vi "Prob.vi"(1 "Data":string[][](array[string])) -> (0 "Success %":dbl, 2 "Histogram_Speed":T1(graph), 3 "Histogram_Length":T1(graph), 4 "E[Speed]":dbl format="%0.2f", 5 "Var[Speed]":dbl format="%0.2f", 6 "E[Length]":dbl format="%0.2f", 7 "Var[Length]":dbl format="%0.2f")   [LabVIEW 2020]
uses:
  <vilib>/Analysis/NI_AALBase.lvlib
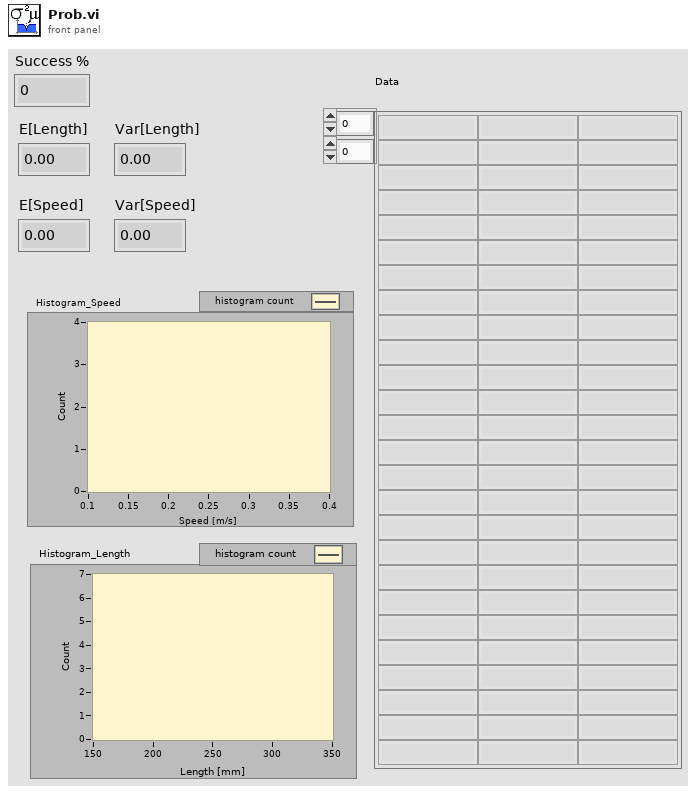
[diagram p1: front panel]
types:
  T1 = cluster{"X Values":dbl[], "Histogram: h(x)":i32[]}
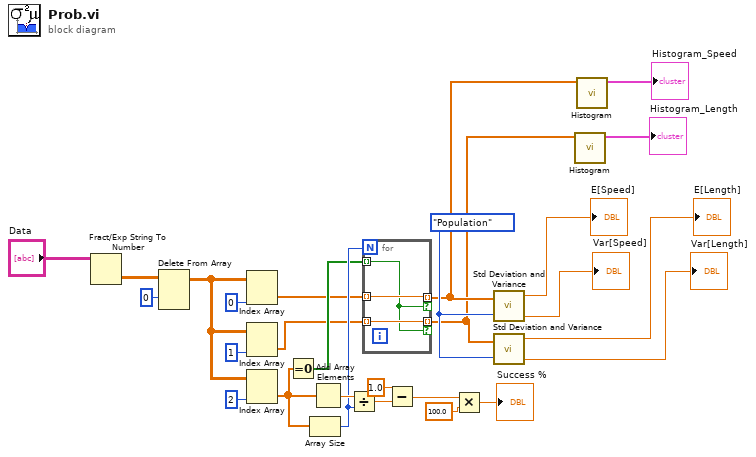
[diagram p0: block diagram]
diagram:
  w7 = enum16{"Sample", "Population"}."Population" ("Weighting (Sample)")
  n1 = Fract/Exp String To Number(string="Data") -> (number=w24:dbl[][])  [unwired: 3 in, 1 out]
  n2 = Delete From Array(array=w24, index (row)=0) -> (array with subset deleted=w21:dbl[][])  [unwired: 2 in, 1 out]
  n3 = Index Array(array=w21, index (col)=0 ("disabled index (col)")) -> (element=w6:dbl[])  [unwired: 1 in]
  n4 = Index Array(array=w21, index (col)=1) -> (element=w12:dbl[])  [unwired: 1 in]
  n5 = Index Array(array=w21, index (col)=2) -> (element=w15:dbl[])  [unwired: 1 in]
  n6 = Equal To 0?(x=w15) -> (x = 0?=w13:bool[])
  n7 = Array Size(array=w15) -> (size(s)=w14:i32)
  n8 = Add Array Elements(numeric array=w15) -> (sum=w22:dbl)
  n9 = Divide(x=w22, y=w14) -> (x/y=w20:dbl)
  n10 = for {
    N: w14 -> [_]
    tunnel: w13 -> [w28] mode=indexing
    tunnel: w6 -> [w30] mode=indexing
    tunnel: w12 -> [w29] mode=indexing
    tunnel: [w30] -> w5 mode=indexing if=w28
    tunnel: [w29] -> w2 mode=indexing if=w28
  }
  n11 = Subtract(x=1.0, y=w20) -> (x-y=w16:dbl)
  n12 = Multiply(x=w16, y=100.0) -> (x*y=→"Success %":dbl)
  n13 = call <vilib>:"Std Deviation and Variance.vi"("X"=w5, "Weighting (Sample)"=w7) -> ("mean"=→"E[Speed]":dbl, "variance"=→"Var[Speed]":dbl)  [unwired: 1 out]
  n14 = call <vilib>:"Std Deviation and Variance.vi"("X"=w2, "Weighting (Sample)"=w7) -> ("mean"=→"E[Length]":dbl, "variance"=→"Var[Length]":dbl)  [unwired: 1 out]
  n15 = call <vilib>:"Histogram.vi"("X"=w2) -> ("Histogram Graph"=→"Histogram_Length":T1)  [unwired: 7 in, 3 out]
  n16 = call <vilib>:"Histogram.vi"("X"=w5) -> ("Histogram Graph"=→"Histogram_Speed":T1)  [unwired: 7 in, 3 out]
